vi "OE1022Dwith BSC.vi"() -> ()   [LabVIEW 2022 SP3]
uses:
  <vilib>/Utility/file.llb/Write Delimited Spreadsheet (string).vi
  <vilib>/Utility/file.llb/Write Delimited Spreadsheet (I64).vi
  <vilib>/Utility/file.llb/Write Delimited Spreadsheet (DBL).vi
  C:/Users/Public/OneDrive/Desktop/PMT program/SampleCodeLabView/Kinesis_with_LabVIEW_Examples_LV12 - v3/Thorlabs.MotionControl.Benchtop.StepperMotorCLI.dll
  PMT program/SampleCodeLabView/Kinesis_with_LabVIEW_Examples_LV12 - v3/Thorlabs.MotionControl.Benchtop.StepperMotorCLI.dll
  C:/Users/Public/OneDrive/Desktop/PMT program/SampleCodeLabView/Kinesis_with_LabVIEW_Examples_LV12 - v3/Thorlabs.MotionControl.GenericMotorCLI.dll
  PMT program/SampleCodeLabView/Kinesis_with_LabVIEW_Examples_LV12 - v3/Thorlabs.MotionControl.GenericMotorCLI.dll
  <vilib>/Analysis/NI_AALBase.lvlib
  C:/Users/Public/OneDrive/Desktop/PMT program/SampleCodeLabView/Kinesis_with_LabVIEW_Examples_LV12 - v3/Thorlabs.MotionControl.Controls.dll
  PMT program/SampleCodeLabView/Kinesis_with_LabVIEW_Examples_LV12 - v3/Thorlabs.MotionControl.Controls.dll
panel:
  in  "SPD":dbl caption="Start Position\nRead Data"
  out "Counter position list":i32[](array[numeric])
  out "mean T":dbl[](array[numeric]) format="%0.2f"
  out "mean list R":dbl[](array[numeric]) format="%0.2f"
  out "Steps Total":i32=2000 caption="Total Steps"
  in  "Range":i32=2000 caption="Range(mm)"
  out "standard deviation T":dbl format="%0.2f"
  out "mean T":dbl format="%0.2f"
  in  "Header":string
  in  "file path (dialog if empty) 2":path
  out "PC":dbl=186.0 caption="Current \nPosition" format="%#_6f"
  in  "SSD":dbl=6.0 caption="Step Size\nRead Data" format="%.4g"
  in  "WT":i32=2000 caption="Wait Time (ms)\n Set Data"
  out "standard deviation R":dbl format="%0.2f"
  in  "Motor Controller\nSerialNumber":string="40837323"
  in  "BenchtopStepperControl":refnum<k24>(container)
  out "Waveform Chart 4":dbl[](graph)=[0.0005999025482049371]
  out "mean R":dbl format="%g"
  out "Waveform Chart 3":dbl[](graph)=[0.0005999025482049371]
  out "θh1 (°) 2":sgl caption="θh1 (deg)" format="%.2f"
  out "Rh1 2":sgl caption="Rh1 (Vrms)" format="%.3p"
  out "Yh1 2":sgl caption="Yh1 (Vrms)" format="%.3p"
  out "Xh1 2":sgl caption="Xh1 (Vrms)" format="%.3p"
  out "Xh2 2":sgl caption="Xh2 (Vrms)" format="%.3p"
  out "Yh2 2":sgl caption="Yh2 (Vrms)" format="%.3p"
  out "Rh2 2":sgl caption="Rh2 (Vrms)" format="%.3p"
  out "噪声 2":sgl caption="Noise(Vrms)" format="%.3p"
  out "频率 (Hz) 2":sgl caption="Freq (Hz)" format="%#.3f"
  out "θ (°) 2":sgl caption="θ (deg)" format="%.2f"
  out "R 2":sgl caption="R (Vrms)" format="%.3p"
  out "Y 2":sgl caption="Y (Vrms)" format="%.3p"
  out "θh2 (°) 2":sgl caption="θh2 (deg)" format="%.2f"
  out "X 2":sgl caption="X (Vrms)" format="%.3p"
  out "Yh1":sgl caption="Yh1 (Vrms)" format="%.3p"
  out "Xh1":sgl caption="Xh1 (Vrms)" format="%.3p"
  out "θh2 (°)":sgl caption="θh2 (deg)" format="%.2f"
  out "Yh2":sgl caption="Yh2 (Vrms)" format="%.3p"
  out "Xh2":sgl caption="Xh2 (Vrms)" format="%.3p"
  out "Rh2":sgl caption="Rh2 (Vrms)" format="%.3p"
  out "θh1 (°)":sgl caption="θh1 (deg)" format="%.2f"
  out "Rh1":sgl caption="Rh1 (Vrms)" format="%.3p"
  out "噪声":sgl caption="Noise(Vrms)" format="%.3p"
  out "频率 (Hz)":sgl caption="Freq (Hz)" format="%#.3f"
  out "θ (°)":sgl caption="θ (deg)" format="%.2f"
  out "Y":sgl caption="Y (Vrms)" format="%.3p"
  out "X":sgl caption="X (Vrms)" format="%.3p"
  out "R":sgl caption="R (Vrms)" format="%.3p"
  out "AUX-ADC2 (V)":sgl format="%.3f"
  out "AUX-ADC1 (V)":sgl format="%.3f"
  out "AUX-ADC3 (V)":sgl format="%.3f"
  out "AUX-ADC4 (V)":sgl format="%.3f"
  out "错误输出":errorcluster
  out "序列号":string
  in  "OE1022D":refnum<visa-resource-name>
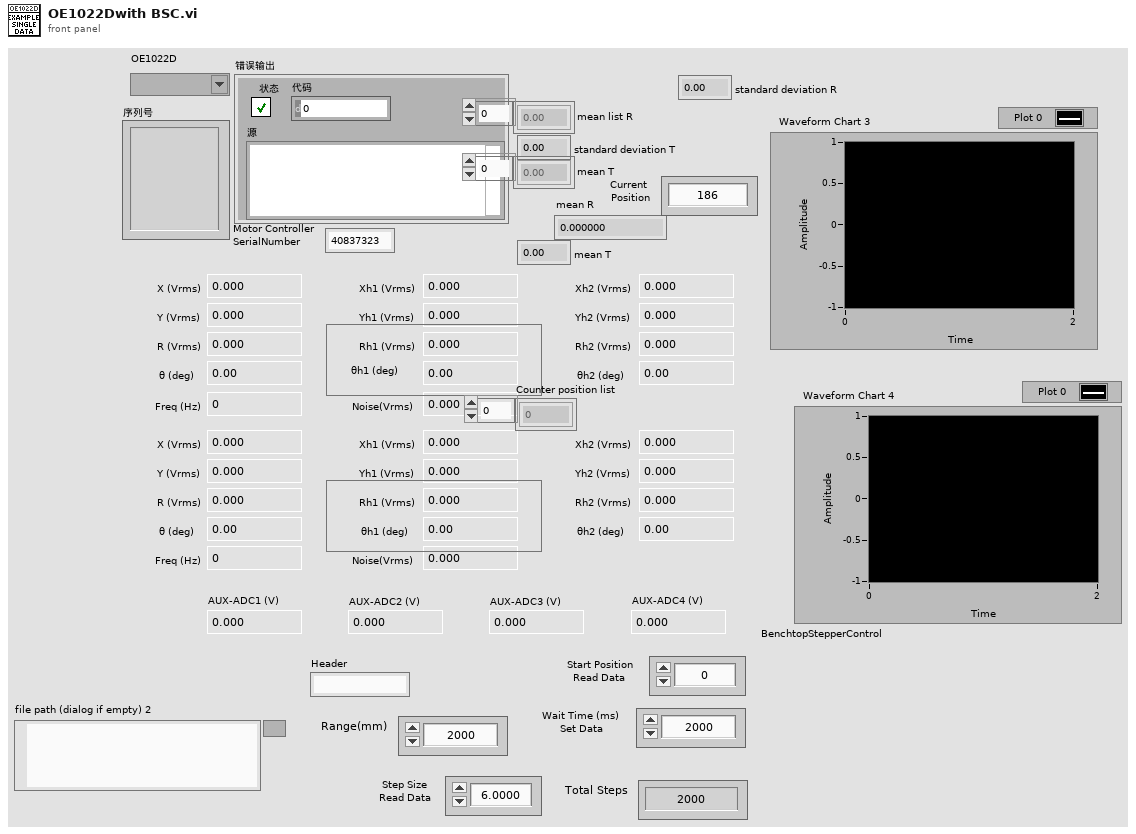
[diagram p1: front panel]
types:
  T1 = cluster{"AD1":dbl[], "AD2":dbl[], "AD3":dbl[], "AD4":dbl[]}
  T2 = cluster{"XB":dbl[], "YB":dbl[], "FrequencyB":dbl[], "NoiseB":dbl[], "Xh1B":dbl[], "Yh1B":dbl[], "Xh2B":dbl[], "Yh2B":dbl[], "Xh2B":dbl[]}
  T3 = cluster{"XA":dbl[], "YA":dbl[], "FrequencyA":dbl[], "NoiseA":dbl[], "Xh1A":dbl[], "Yh1A":dbl[], "Xh2A":dbl[], "Yh2A":dbl[]}
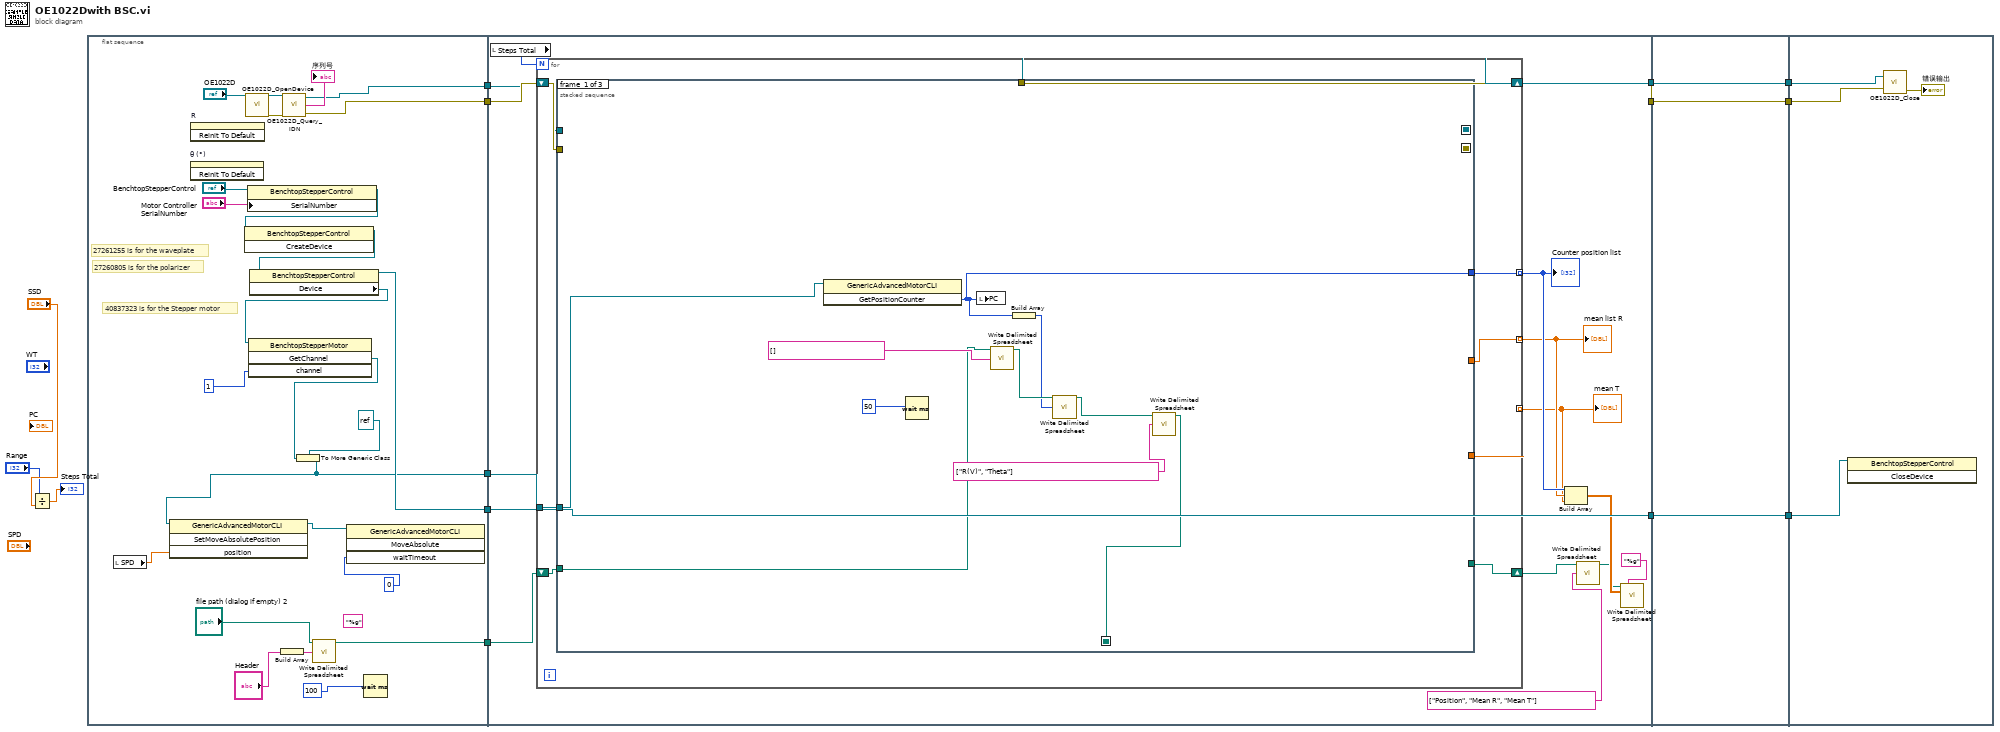
[diagram p0: block diagram]
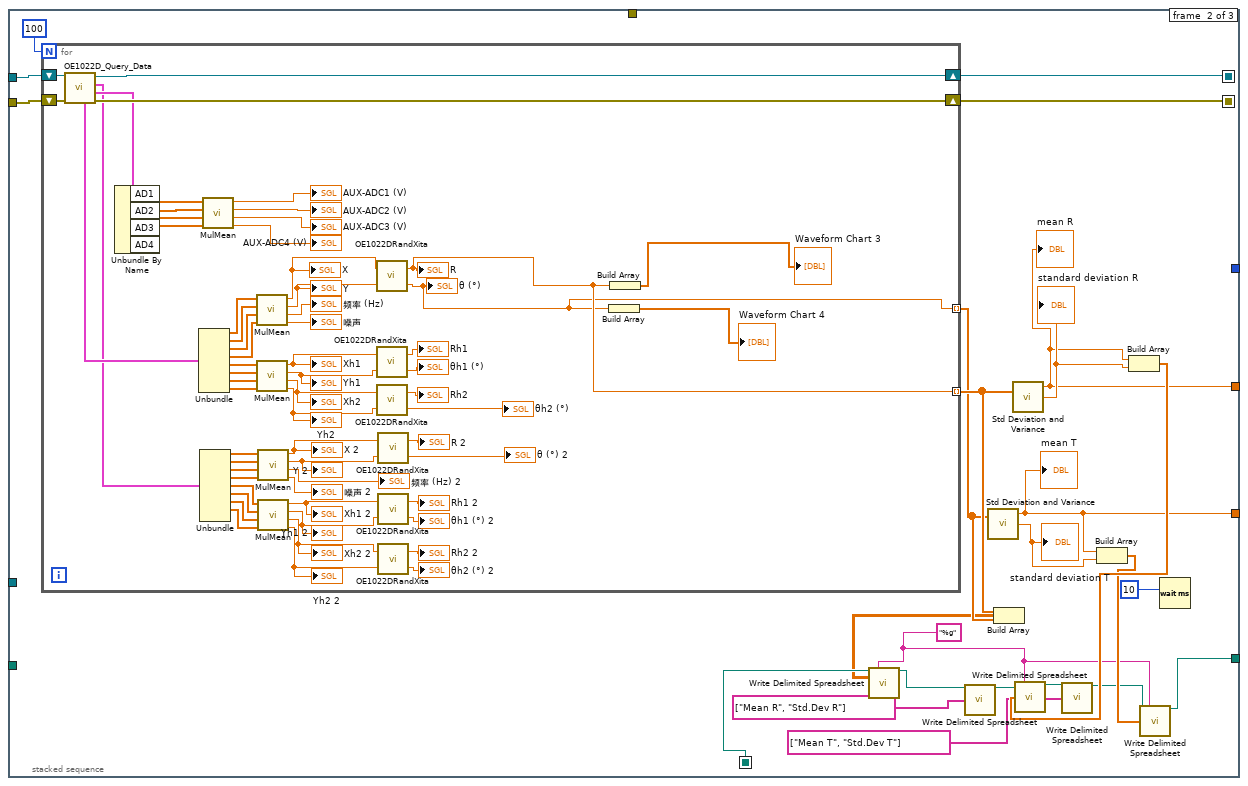
[diagram p2: hidden frame]
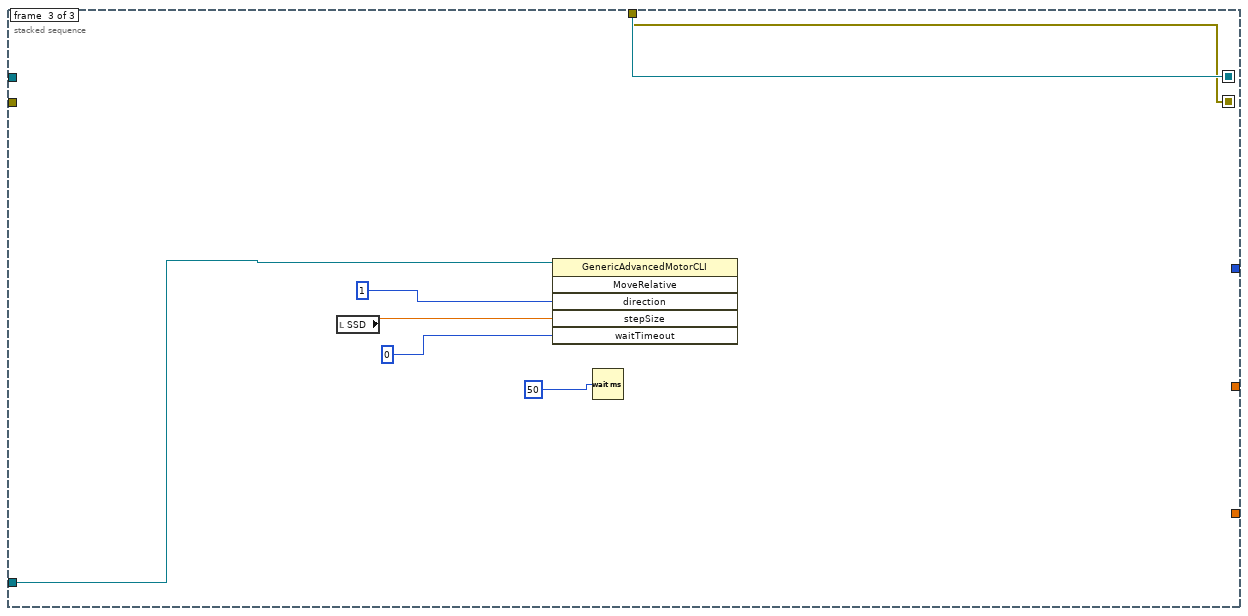
[diagram p3: hidden frame]
diagram:
  n1 = Divide(x="Range", y="SSD") -> (x/y=→"Steps Total":dbl)
  n2 = flat-sequence {
    tunnel: [w34] -> w14
    tunnel: [w33] -> w13
    tunnel: [w23] -> w6
    tunnel: [w18] -> w5
    tunnel: [w19] -> w4
    tunnel: w14 -> [w54]
    tunnel: w13 -> [w51]
    tunnel: [w53] -> w12
    tunnel: [w52] -> w11
    tunnel: [w50] -> w7
    tunnel: w6 -> [w50]
    tunnel: w5 -> [w49]
    tunnel: w4 -> [w39]
    tunnel: w12 -> [w169]
    tunnel: [w169] -> w10
    tunnel: w11 -> [w168]
    tunnel: [w168] -> w9
    tunnel: [w167] -> w8
    tunnel: w7 -> [w167]
    tunnel: w10 -> [w171]
    tunnel: w9 -> [w172]
    tunnel: w8 -> [w170]
    frame #0 {
      (unwired) "%g" ("format (%.3f)")
      # "40837323 is for the Stepper motor"
      # "27260805 is for the polarizer"
      # "27261255 is for the waveplate"
      n3 = local read "SPD"() -> (w16:dbl)
      n4 = invoke on="θ (°)" class="DigNum (strict)" method="Reinit To Default"() -> ()  [unwired: 3 in, 3 out]
      n5 = invoke on="R" class="DigNum (strict)" method="Reinit To Default"() -> ()  [unwired: 3 in, 3 out]
      n6 = call "OE1022D_OpenDevice.vi"("VISA resource name"="OE1022D") -> ("VISA资源名称输出"=w35:refnum<visa-resource-name>, "错误输出"=w37:errorcluster)  [unwired: 17 in]
      n7 = property class="BenchtopStepperControl"(reference="BenchtopStepperControl", "SerialNumber"="Motor Controller\nSerialNumber") -> (reference out=w28:refnum<k24>)  [unwired: 1 in, 1 out]
      n8 = invoke class="BenchtopStepperControl" method="CreateDevice"(reference=w28) -> (reference out=w30:refnum<k24>)  [unwired: 2 in, 2 out]
      n9 = property class="BenchtopStepperControl"(reference=w30) -> (reference out=w23:refnum<k24>, "Device"=w31:refnum<k24>)  [unwired: 1 in, 1 out]
      n10 = invoke class="BenchtopStepperMotor" method="GetChannel"(reference=w31, "channel"=1) -> ("GetChannel"=w32:refnum<k24>)  [unwired: 2 in, 3 out]
      n11 = Build Array("Header") -> (w20:string[])
      n12 = call "OE1022D_Query_IDN.vi"("错误输入（无错误）"=w37, "VISA resource name"=w35) -> ("错误输出"=w34:errorcluster, "序列号"=→"序列号":string, "VISA resource name out"=w33:refnum<visa-resource-name>)  [unwired: 1 in]
      n13 = To More Generic Class(target class=refnum<k24> refnum, reference=w32) -> (generic class reference=w18:refnum<k24>)
      n14 = invoke class="GenericAdvancedMotorCLI" method="SetMoveAbsolutePosition"(reference=w18, "position"=w16) -> (reference out=w17:refnum<k24>)  [unwired: 2 in, 3 out]
      n15 = call-poly <vilib>:"Write Delimited Spreadsheet.vi"("file path (dialog if empty)"="file path (dialog if empty) 2", "1D data"=w20) -> ("new file path (Not A Path if cancelled)"=w19:path)  [unwired: 12 in, 1 out]
      n16 = invoke class="GenericAdvancedMotorCLI" method="MoveAbsolute"(reference=w17, "waitTimeout"=0) -> ()  [unwired: 2 in, 4 out]
      n17 = Wait (ms)(milliseconds to wait=100) -> ()  [unwired: 1 out]
    }
    frame #1 {
      n18 = local read "Steps Total"() -> (w48:i32)
      n19 = for {
        N: w48 -> [_]
        tunnel: w49 -> [w60]
        shift-right: [w62] -> w52
        shift-left: w54 -> [w64]
        shift-right: [w63] -> w53
        shift-left: w51 -> [w61]
        tunnel: [w59] -> w44 mode=indexing
        tunnel: [w58] -> w43 mode=indexing
        tunnel: [w57] -> w45 mode=indexing
        shift-right: [w56] -> w47
        shift-left: w39 -> [w55]
        n20 = stacked-sequence {
          seq-local: [_ w97 _] -> [_ _ w166]
          seq-local: [_ w96 _] -> [_ _ w165]
          seq-local: [w68 _ _] -> [_ w93 _]
          tunnel: w64 -> [_ w98 _]
          tunnel: w61 -> [_ w95 _]
          tunnel: [_ _ w166] -> w63
          tunnel: [_ _ w165] -> w62
          tunnel: w60 -> [w74 _ w162]
          tunnel: [_ w77 _] -> w59
          tunnel: [_ w76 _] -> w58
          tunnel: [w66 _ _] -> w57
          tunnel: [_ w75 _] -> w56
          tunnel: w55 -> [w65 _ _]
          frame #0 {
            n21 = invoke class="GenericAdvancedMotorCLI" method="GetPositionCounter"(reference=w74) -> ("GetPositionCounter"=w66:i32)  [unwired: 2 in, 2 out]
            n22 = Wait (ms)(milliseconds to wait=50) -> ()  [unwired: 1 out]
            n23 = local write "PC"(w66) -> ()
            n24 = call-poly <vilib>:"Write Delimited Spreadsheet.vi"("file path (dialog if empty)"=w65, "1D data"=string[] []) -> ("new file path (Not A Path if cancelled)"=w71:path)  [unwired: 12 in, 1 out]
            n25 = Build Array(w66) -> (w70:i32[])
            n26 = call-poly <vilib>:"Write Delimited Spreadsheet.vi"("file path (dialog if empty)"=w71, "1D data"=w70) -> ("new file path (Not A Path if cancelled)"=w69:path)  [unwired: 12 in, 1 out]
            n27 = call-poly <vilib>:"Write Delimited Spreadsheet.vi"("file path (dialog if empty)"=w69, "1D data"=string[] ["R(V)", "Theta"]) -> ("new file path (Not A Path if cancelled)"=w68:path)  [unwired: 12 in, 1 out]
          }
          frame #1 {
            w78 = "%g" ("format (%.3f)")
            n28 = for {
              N: 100 -> [_]
              shift-right: [w157] -> w96
              shift-left: w98 -> [w159]
              shift-right: [w158] -> w97
              shift-left: w95 -> [w156]
              tunnel: [w101] -> w91 mode=indexing
              tunnel: [w99] -> w90 mode=indexing
              n29 = call "OE1022D_Query_Data.vi"("错误输入（无错误）"=w159, "VISA resource name"=w156) -> ("error out"=w157:errorcluster, "输出簇ADC"=w108:T1, "输出簇B"=w107:T2, "VISA resource name out"=w158:refnum<visa-resource-name>, "输出簇A"=w109:T3)  [unwired: 3 in]
              n30 = Unbundle By Name(w108) -> ("AD1"=w152:dbl[], "AD2"=w153:dbl[], "AD3"=w154:dbl[], "AD4"=w155:dbl[])
              n31 = Unbundle(w109) -> ("XA"=w114:dbl[], "YA"=w115:dbl[], "FrequencyA"=w116:dbl[], "NoiseA"=w117:dbl[], "Xh1A"=w122:dbl[], "Yh1A"=w123:dbl[], "Xh2A"=w124:dbl[], "Yh2A"=w125:dbl[])
              n32 = Unbundle(w107) -> ("XB"=w139:dbl[], "YB"=w138:dbl[], "FrequencyB"=w137:dbl[], "NoiseB"=w136:dbl[], "Xh1B"=w135:dbl[], "Yh1B"=w134:dbl[], "Xh2B"=w133:dbl[], "Yh2B"=w132:dbl[])  [unwired: 1 out]
              n33 = call "MulMean.vi"("IN 4"=w155, "IN 3"=w154, "IN 2"=w153, "IN 1"=w152) -> ("mean 4"=→"AUX-ADC4 (V)":dbl, "mean 3"=→"AUX-ADC3 (V)":dbl, "mean 2"=→"AUX-ADC2 (V)":dbl, "mean 1"=→"AUX-ADC1 (V)":dbl)  [unwired: 4 in]
              n34 = call "MulMean.vi"("IN 4"=w117, "IN 3"=w116, "IN 2"=w115, "IN 1"=w114) -> ("mean 4"=→"噪声":dbl, "mean 3"=→"频率 (Hz)":dbl, "mean 2"=w120:dbl, "mean 1"=w119:dbl)  [unwired: 4 in]
              "X" <- w119
              "Y" <- w120
              n35 = call "MulMean.vi"("IN 4"=w125, "IN 3"=w124, "IN 2"=w123, "IN 1"=w122) -> ("mean 4"=w129:dbl, "mean 3"=w128:dbl, "mean 2"=w127:dbl, "mean 1"=w126:dbl)  [unwired: 4 in]
              "Xh2" <- w128
              "Yh2" <- w129
              "Xh1" <- w126
              "Yh1" <- w127
              n36 = call "MulMean.vi"("IN 4"=w136, "IN 3"=w137, "IN 2"=w138, "IN 1"=w139) -> ("mean 4"=→"噪声 2":dbl, "mean 3"=→"频率 (Hz) 2":dbl, "mean 2"=w145:dbl, "mean 1"=w144:dbl)  [unwired: 4 in]
              "X 2" <- w144
              "Y 2" <- w145
              n37 = call "MulMean.vi"("IN 4"=w132, "IN 3"=w133, "IN 2"=w134, "IN 1"=w135) -> ("mean 4"=w149:dbl, "mean 3"=w148:dbl, "mean 2"=w147:dbl, "mean 1"=w146:dbl)  [unwired: 4 in]
              "Yh2 2" <- w149
              "Xh2 2" <- w148
              "Xh1 2" <- w146
              "Yh1 2" <- w147
              n38 = call "OE1022DRandXita.vi"("Y"=w120, "X"=w119) -> ("θ (°)"=w99:dbl, "R"=w101:dbl)
              "R" <- w101
              "θ (°)" <- w99
              n39 = call "OE1022DRandXita.vi"("Y"=w127, "X"=w126) -> ("θ (°)"=→"θh1 (°)":dbl, "R"=→"Rh1":dbl)
              n40 = call "OE1022DRandXita.vi"("Y"=w129, "X"=w128) -> ("θ (°)"=→"θh2 (°)":dbl, "R"=→"Rh2":dbl)
              n41 = call "OE1022DRandXita.vi"("Y"=w145, "X"=w144) -> ("θ (°)"=→"θ (°) 2":dbl, "R"=→"R 2":dbl)
              n42 = call "OE1022DRandXita.vi"("Y"=w147, "X"=w146) -> ("θ (°)"=→"θh1 (°) 2":dbl, "R"=→"Rh1 2":dbl)
              n43 = call "OE1022DRandXita.vi"("Y"=w149, "X"=w148) -> ("θ (°)"=→"θh2 (°) 2":dbl, "R"=→"Rh2 2":dbl)
              n44 = Build Array(w99) -> (→"Waveform Chart 4":dbl[])
              n45 = Build Array(w101) -> (→"Waveform Chart 3":dbl[])
            }
            n46 = call <vilib>:"Std Deviation and Variance.vi"("X"=w90) -> ("mean"=w76:dbl, "standard deviation"=w81:dbl)  [unwired: 1 in, 1 out]
            "mean T" <- w76
            "standard deviation T" <- w81
            n47 = Build Array(w91, w90) -> (w89:dbl[][])
            n48 = call-poly <vilib>:"Write Delimited Spreadsheet.vi"("file path (dialog if empty)"=w93, "format (%.3f)"=w78, "2D data"=w89) -> ("new file path (Not A Path if cancelled)"=w88:path)  [unwired: 11 in, 1 out]
            n49 = call-poly <vilib>:"Write Delimited Spreadsheet.vi"("file path (dialog if empty)"=w88, "1D data"=string[] ["Mean R", "Std.Dev R"] ("format (%.3f)")) -> ("new file path (Not A Path if cancelled)"=w86:path)  [unwired: 12 in, 1 out]
            n50 = call <vilib>:"Std Deviation and Variance.vi"("X"=w91) -> ("mean"=w77:dbl, "standard deviation"=w85:dbl)  [unwired: 1 in, 1 out]
            "mean R" <- w77
            "standard deviation R" <- w85
            n51 = Build Array(w76, w81) -> (w80:dbl[])
            n52 = Build Array(w77, w85) -> (w84:dbl[])
            n53 = call-poly <vilib>:"Write Delimited Spreadsheet.vi"("file path (dialog if empty)"=w86, "format (%.3f)"=w78, "1D data"=w84) -> ("new file path (Not A Path if cancelled)"=w82:path)  [unwired: 11 in, 1 out]
            n54 = call-poly <vilib>:"Write Delimited Spreadsheet.vi"("file path (dialog if empty)"=w82, "1D data"=string[] ["Mean T", "Std.Dev T"] ("format (%.3f)")) -> ("new file path (Not A Path if cancelled)"=w79:path)  [unwired: 12 in, 1 out]
            n55 = call-poly <vilib>:"Write Delimited Spreadsheet.vi"("file path (dialog if empty)"=w79, "format (%.3f)"=w78, "1D data"=w80) -> ("new file path (Not A Path if cancelled)"=w75:path)  [unwired: 11 in, 1 out]
            n56 = Wait (ms)(milliseconds to wait=10) -> ()  [unwired: 1 out]
          }
          frame #2 {
            n57 = local read "SSD"() -> (w160:dbl)
            n58 = invoke class="GenericAdvancedMotorCLI" method="MoveRelative"(reference=w162, "direction"=1, "stepSize"=w160, "waitTimeout"=0) -> ()  [unwired: 2 in, 6 out]
            n59 = Wait (ms)(milliseconds to wait=50) -> ()  [unwired: 1 out]
          }
        }
      }
      "mean list R" <- w44
      "mean T" <- w43
      "Counter position list" <- w45
      n60 = Build Array(w45, w44, w43) -> (w42:dbl[][])
      n61 = call-poly <vilib>:"Write Delimited Spreadsheet.vi"("file path (dialog if empty)"=w47, "1D data"=string[] ["Position", "Mean R", "Mean T"] ("format (%.3f)")) -> ("new file path (Not A Path if cancelled)"=w41:path)  [unwired: 12 in, 1 out]
      n62 = call-poly <vilib>:"Write Delimited Spreadsheet.vi"("file path (dialog if empty)"=w41, "format (%.3f)"="%g", "2D data"=w42) -> ()  [unwired: 11 in, 2 out]
    }
    frame #2 {
    }
    frame #3 {
      n63 = invoke class="BenchtopStepperControl" method="CloseDevice"(reference=w170) -> ()  [unwired: 2 in, 3 out]
      n64 = call "OE1022D_Close.vi"("错误输入（无错误）"=w172, "VISA resource name"=w171) -> ("错误输出"=→"错误输出":errorcluster)  [unwired: 1 in]
    }
  }
